vi "PathDrawerMain.vi"() -> ()   [LabVIEW 2018]
uses:
  StartingPositions.ctl
  Dawgma Programming Library/Controls/PurePursuit/PathFileData.ctl
  Dawgma Programming Library/Controls/PurePursuit/RobotNeededPathData.ctl
  <vilib>/Utility/miscctls.llb/LVBoundsTypeDef.ctl
  Robot-Project/Configuration/Constants.vi
panel:
  in  "NoUpdate":bool
  out "PathsStorage":T1[](array[typedef])=[{"RobotNeeded"={"Path"=[{67.51826792963463, 204.30852503382948}, {73.33752695702532, 204.17640783242763}, {79.12917348553499, 204.07996681682357}, {84.86117778762187, 204.06061787570727}, {90.49184817844007, 204.17225057986516}, {95.96307089902717, 204.48997502749893}, {101.19090415563274, 205.12228366964248}, {106.05199464247043, 206.2286051295332}, {110.36361644562574, 208.04511161169543}, {114.37172578385798, 210.89248691926605}, {118.17642408641785, 214.43024981480622}, {121.84478802267412, 218.4296155778484}, {125.42197657870013, 222.73663853194364}, {128.93822516173634, 227.24710298781127}, {132.4139659676452, 231.88974137154145}, {135.8631515190472, 236.6147503980893}, {139.2952430485304, 241.3855785202741}, {142.71714395845063, 246.1731860201357}, {146.13394637043862, 250.9511479319172}, {149.5499982146016, 255.691538218544}, {152.9695484837296, 260.36036298292}, {156.39736200192732, 264.9119963112372}, {159.8395350266317, 269.28183564054643}, {163.30451800782737, 273.375872369032}, {166.80445999957857, 277.0554498679603}, {170.3571607758867, 280.1148018612651}, {174.375619494585, 282.81240477743506}, {178.60376106475013, 285.2362954814753}, {182.8194665712848, 287.43019005020165}, {186.79860760663416, 289.40056942324793}, {190.27875507442488, 291.11772665764545}], "MaxVel"=150.0, "MaxAccel"=150.0, "Backwards?"=FALSE, "PointSpacing"=6.0, "LookaheadDist"=17.0, "Speed/Curve"=3.0, "SlowDistanceAtEnd"=0.0, "SlowSpeed"=15.0, "MaxDeAccel"=120.0}, "Meta"={"Path (px)"=[{97, 141}, {148, 144}, {211, 52}, {237, 42}], "RobotWidth"=33.0, "RobotLength"=38.5, "CenterOfRotYOffset"=19.5, "Roundedness"=0.8606565656565657, "StartingPositionPreset"=0}}] {"RobotNeeded"."SlowSpeed" format="%#_13g"; "RobotNeeded"."SlowDistanceAtEnd" format="%#_13g"; "RobotNeeded"."Speed/Curve" format="%#_13g"}
  in  "Tab Control":enum32{"Path", "Load/Save"}(tab)
  in  "SetStart":bool
  in  "Deaccel":dbl=120.0 format="%#_13g"
  in  "SlowSpeed":dbl=15.0 format="%#_13g"
  in  "SlowDistanceAtEnd":dbl format="%#_13g"
  in  "Speed/Curve":dbl=3.0 format="%#_13g"
  in  "DriveBackwards?":bool
  in  "Lookahead":dbl=17.0
  in  "Points (in)":cluster{dbl, dbl}[](array[cluster])=[{67.51826792963463, 204.30852503382948}, {73.33752695702532, 204.17640783242763}, {79.12917348553499, 204.07996681682357}, {84.86117778762187, 204.06061787570727}, {90.49184817844007, 204.17225057986516}, {95.96307089902717, 204.48997502749893}, {101.19090415563274, 205.12228366964248}, {106.05199464247043, 206.2286051295332}, {110.36361644562574, 208.04511161169543}, {114.37172578385798, 210.89248691926605}, {118.17642408641785, 214.43024981480622}, {121.84478802267412, 218.4296155778484}, {125.42197657870013, 222.73663853194364}, {128.93822516173634, 227.24710298781127}, {132.4139659676452, 231.88974137154145}, {135.8631515190472, 236.6147503980893}, {139.2952430485304, 241.3855785202741}, {142.71714395845063, 246.1731860201357}, {146.13394637043862, 250.9511479319172}, {149.5499982146016, 255.691538218544}, {152.9695484837296, 260.36036298292}, {156.39736200192732, 264.9119963112372}, {159.8395350266317, 269.28183564054643}, {163.30451800782737, 273.375872369032}, {166.80445999957857, 277.0554498679603}, {170.3571607758867, 280.1148018612651}, {174.375619494585, 282.81240477743506}, {178.60376106475013, 285.2362954814753}, {182.8194665712848, 287.43019005020165}, {186.79860760663416, 289.40056942324793}, {190.27875507442488, 291.11772665764545}]
  out "Points (px)":cluster{dbl, dbl}[](array[cluster])=[{97.0, 141.0}, {148.0, 144.0}, {211.0, 52.0}, {237.0, 42.0}]
  in  "Roundedness":dbl(slide)=0.8606565656565657 scale=0.6..0.997
  in  "PointSpacing":dbl=6.0 min=1.0 format="%#_13g"
  in  "Flip Path":bool
  in  "MaxVel":dbl=150.0 format="%#_13g"
  in  "Accel":dbl=150.0 format="%#_13g"
  in  "StartingPosition":T3
  in  "Multiple Paths":i32(listbox)
  in  "ExportAllToRobot":bool
  in  "LocalTempPaths":i32(listbox)
  out "standard output":string
  in  "SaveToLocal":bool
  in  "LoadFromLocal":bool
  in  "ExportToRobot":bool
  in  "LoadAllFromRobot":bool
  in  "LocalPaths":i32(listbox)
  out "standard error":string="NI Linux Real-Time (run mode)\n\nLog in with your NI-Auth credentials.\n\n"
  in  "LocalFileNames":string[](array[string])=["1LL.txt", "3RR.txt"]
  out "Path Drawer":T4(plugin-control)
  # "(Double Click)"
  # "INSTRUCTIONS"
  # "The red line is the path that the robot recieves. Everything else is to help create that path\n\nUse the multi-line tool to draw a path. Double click to stop drawing.\nHover over a node and press backspace to remove it.\nPress I to insert a new node (at the end of the path only, for now)\n\nUse the contols to input robot width, height, and center of rotation offset,\nHow far apart the points in the \"real world units\" path are,\nWhether the robot travels on the left or right of your green lines, and\nthe roundedness of the path. (Note: point spacing affects roundedness)\n\nYou can manually edit the green node's location in the path with the Points array,\nor drag the nodes on the image\n\nPress Export To File and enter the file name (no extension) to save the path to a file in the\nThisVIsDirectory\\Paths\\ folder\n\nIf you acidentally clear your path press Z quickly to get it back"
  # "Responses of CMDs run"
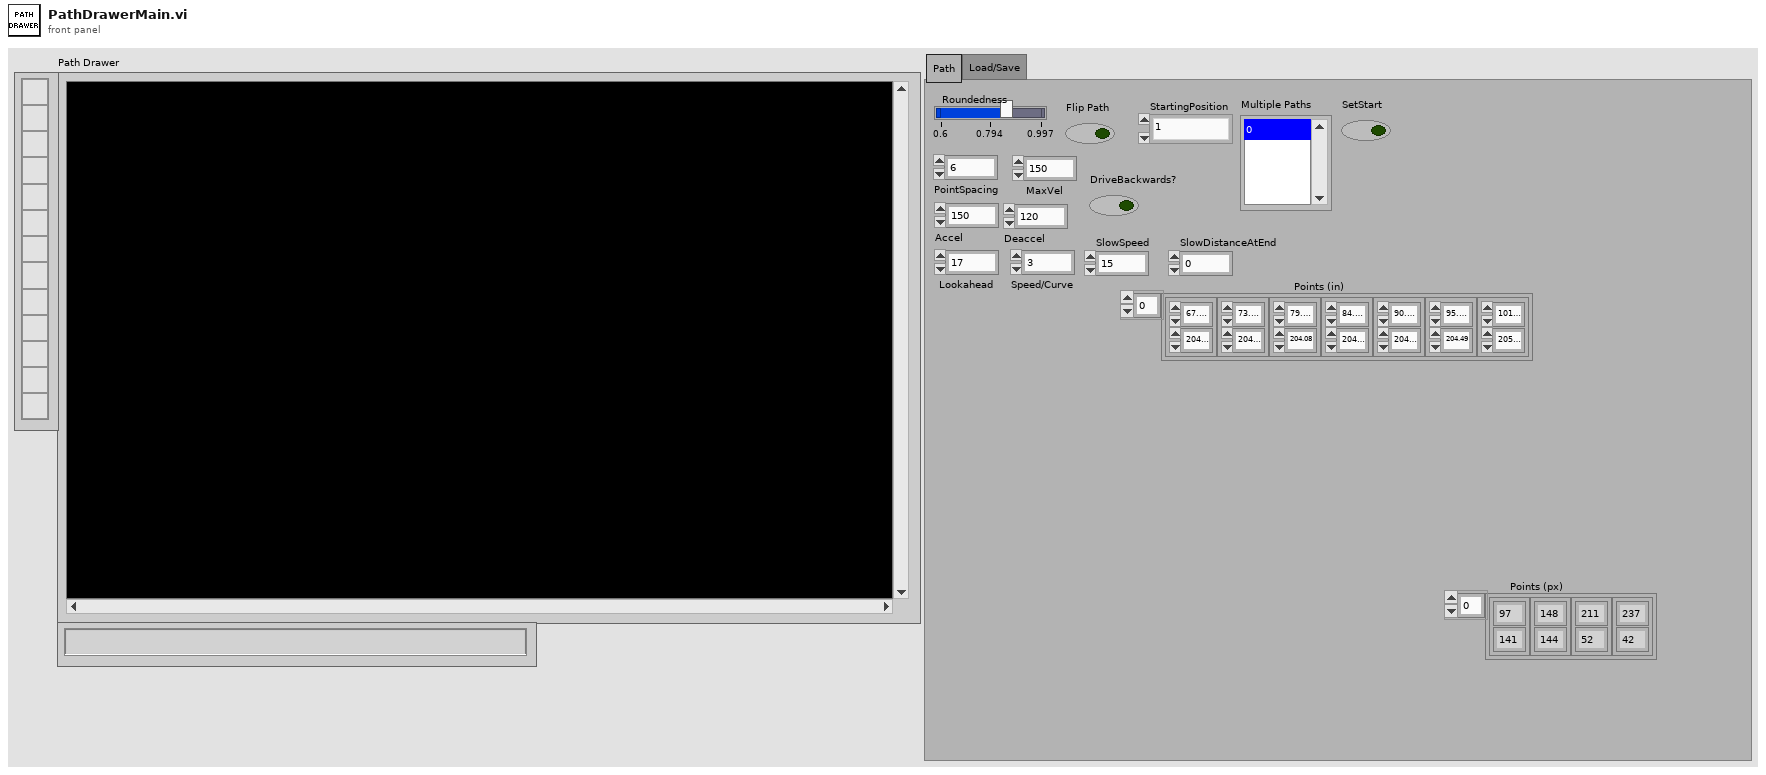
[diagram p1: front panel]
types:
  T1 = typedef "PathFileData.ctl" = cluster{"RobotNeeded":T2, "Meta":cluster{"Path (px)":cluster{i32, i32}[], "RobotWidth":dbl, "RobotLength":dbl, "CenterOfRotYOffset":dbl, "Roundedness":dbl, "StartingPositionPreset":u32}}
  T2 = typedef "RobotNeededPathData.ctl" = cluster{"Path":cluster{dbl, dbl}[], "MaxVel":dbl, "MaxAccel":dbl, "Backwards?":bool, "PointSpacing":dbl, "LookaheadDist":dbl, "Speed/Curve":dbl, "SlowDistanceAtEnd":dbl, "SlowSpeed":dbl, "MaxDeAccel":dbl}
  T3 = typedef "StartingPositions.ctl" = enum16{"1", "2", "3", "4", "5", "No Preset"}
  T4 = typedef "IMAQ Image.ctl" = refnum<image>
  T5 = typedef "Image Type" = u32
  T6 = enum16{"open", "replace", "create", "open or create", "replace or create", "replace or create with confirmation"}
  T7 = typedef "LVBoundsTypeDef.ctl" = cluster{"Width":u32, "Height":u32}
  T8 = cluster{"Global Rectangle":i32[], "Contours":cluster{"Contour Type":u32, "ROI Type":u32, "Points":i32[]}[]}
  T9 = cluster{"Contour Type":u32, "ROI Type":u32, "Points":i32[]}[]
  T10 = cluster{"Contour Type":u32, "ROI Type":u32, "Points":i32[]}
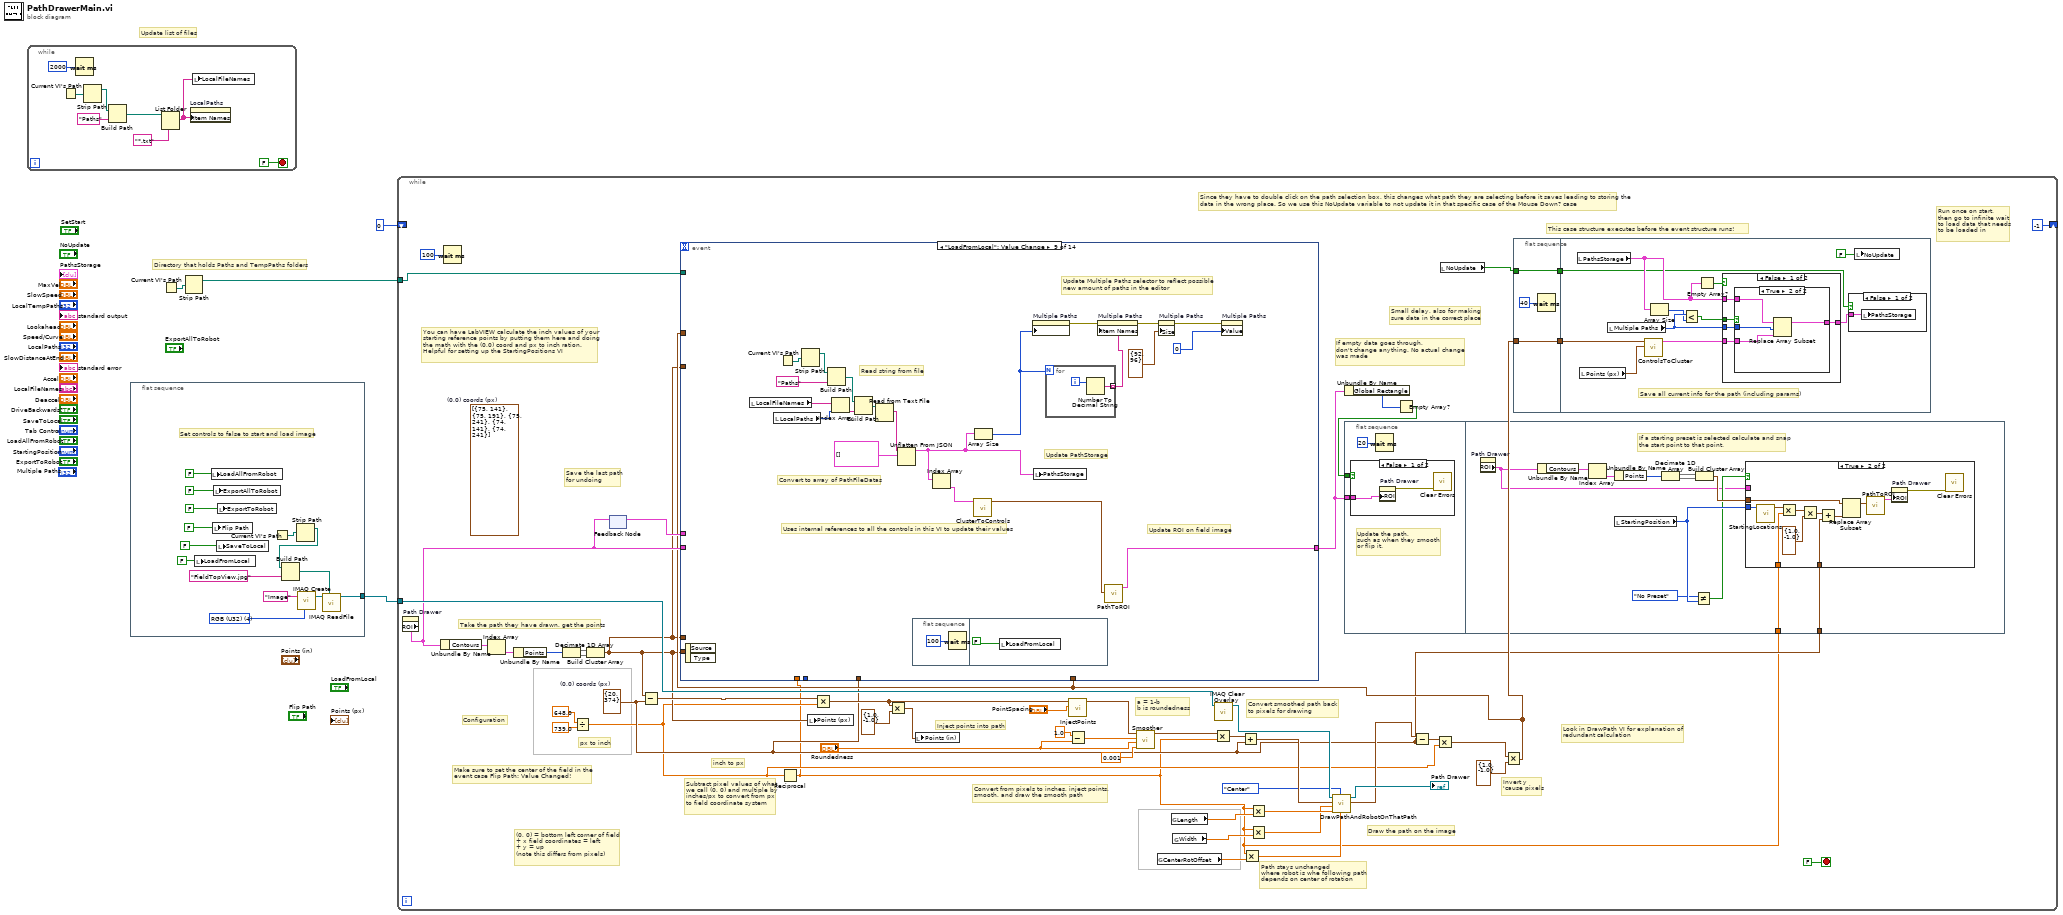
[diagram p0: block diagram]
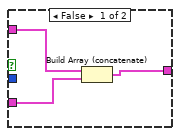
[diagram p3: hidden frame]
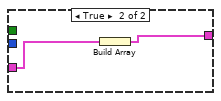
[diagram p4: hidden frame]
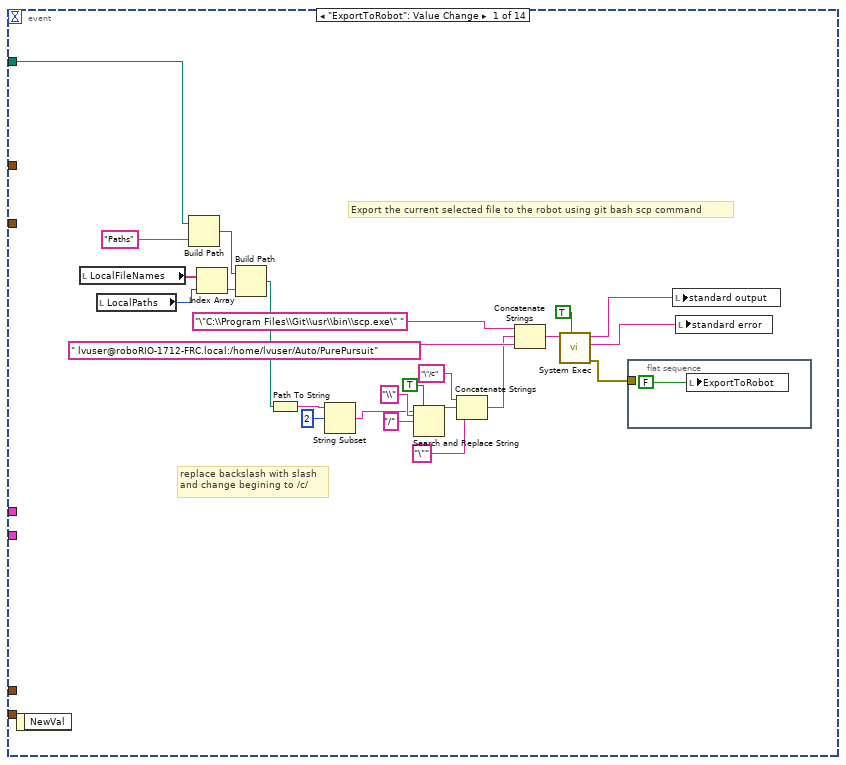
[diagram p7: hidden frame]
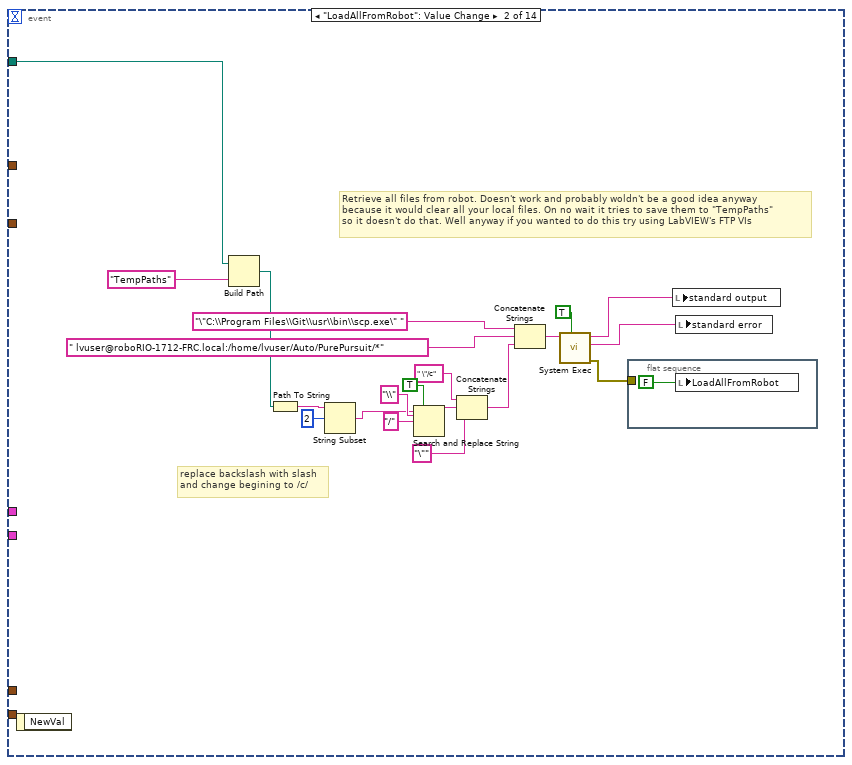
[diagram p8: hidden frame]
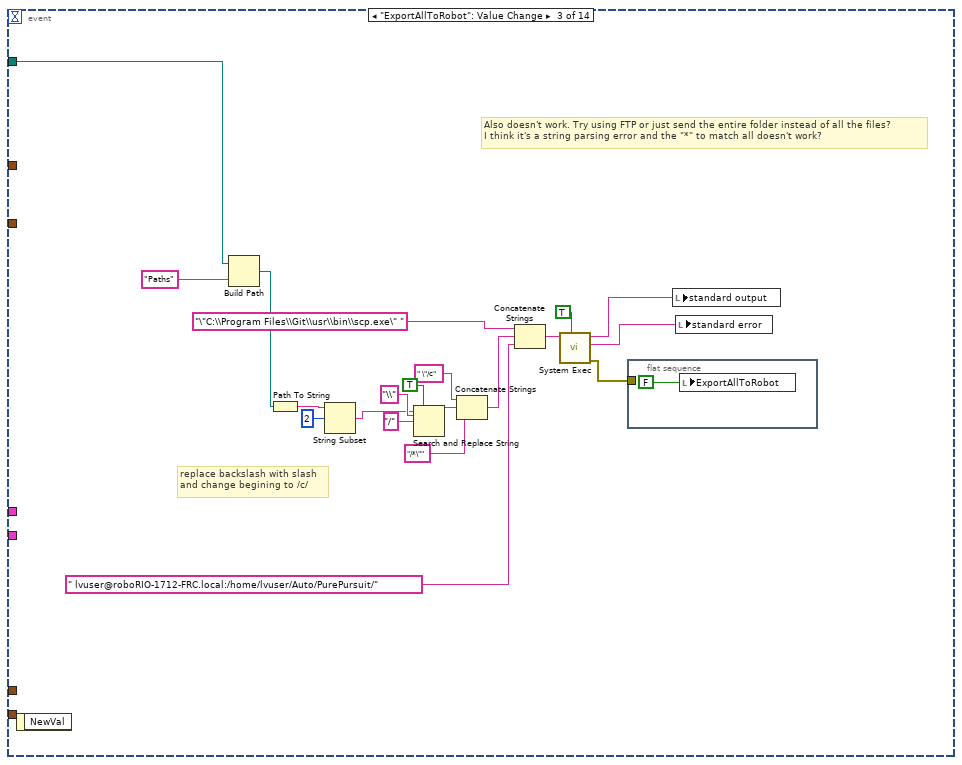
[diagram p9: hidden frame]
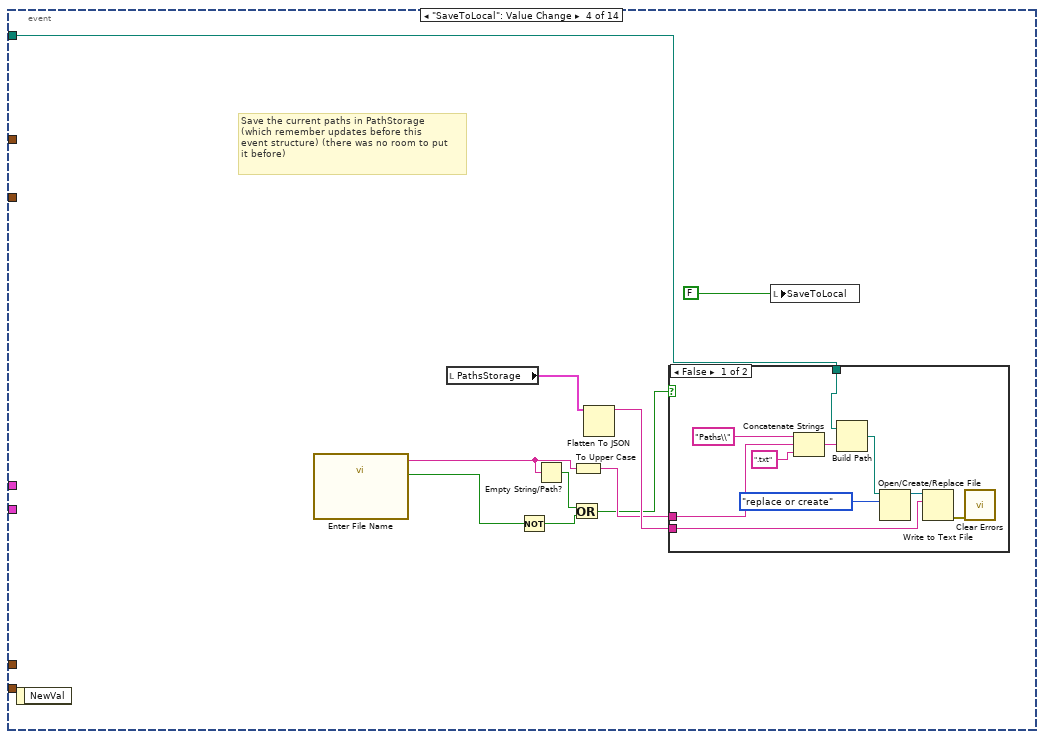
[diagram p10: hidden frame]
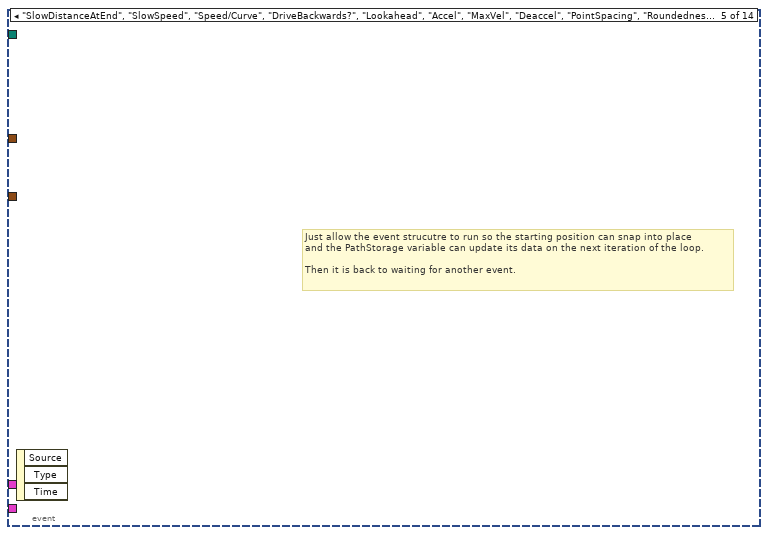
[diagram p12: hidden frame]
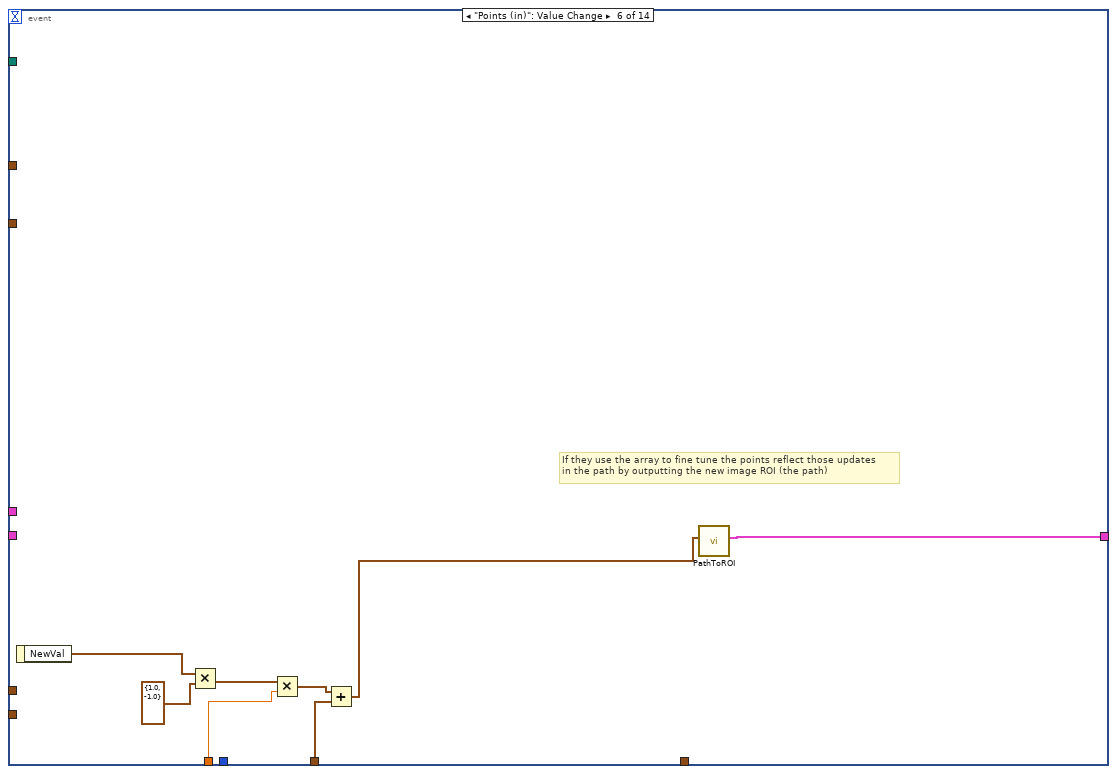
[diagram p13: hidden frame]
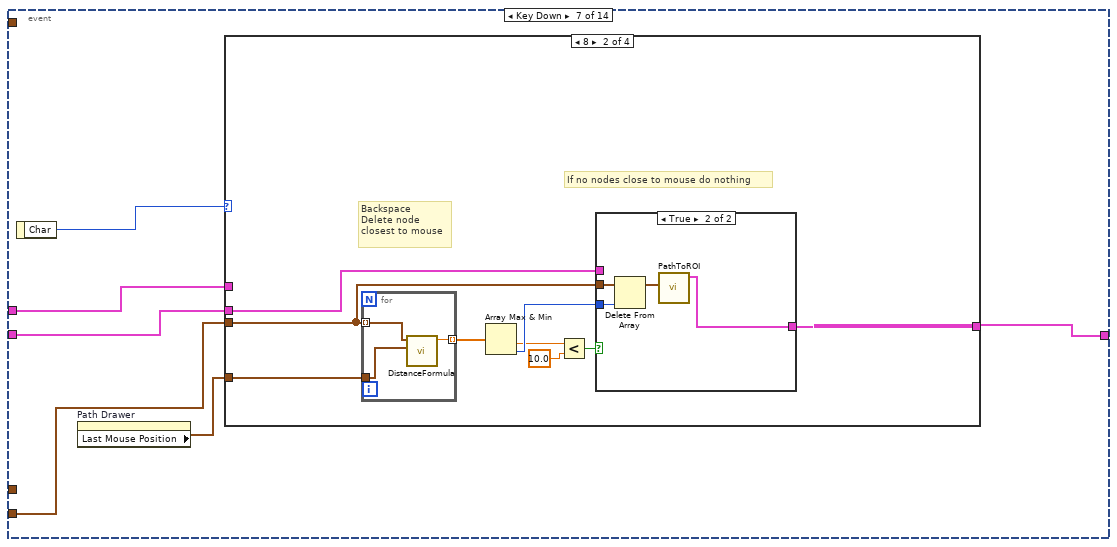
[diagram p14: hidden frame]
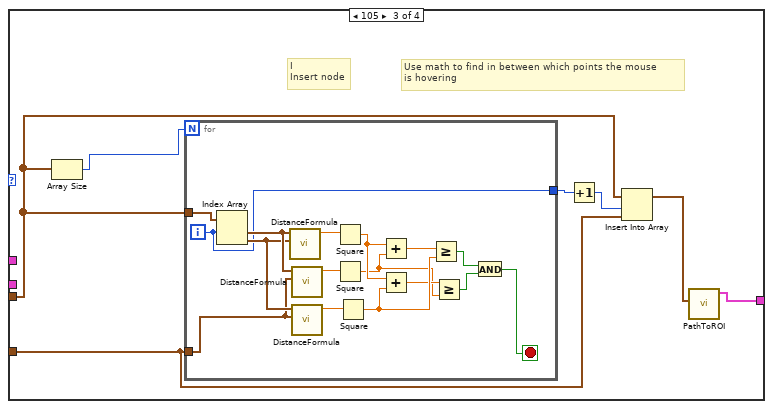
[diagram p17: hidden frame]
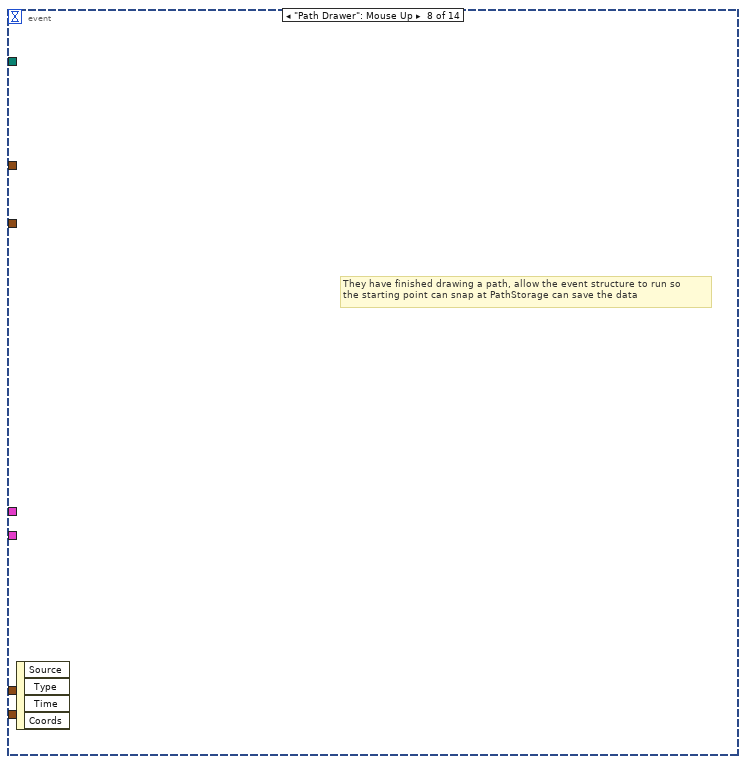
[diagram p19: hidden frame]
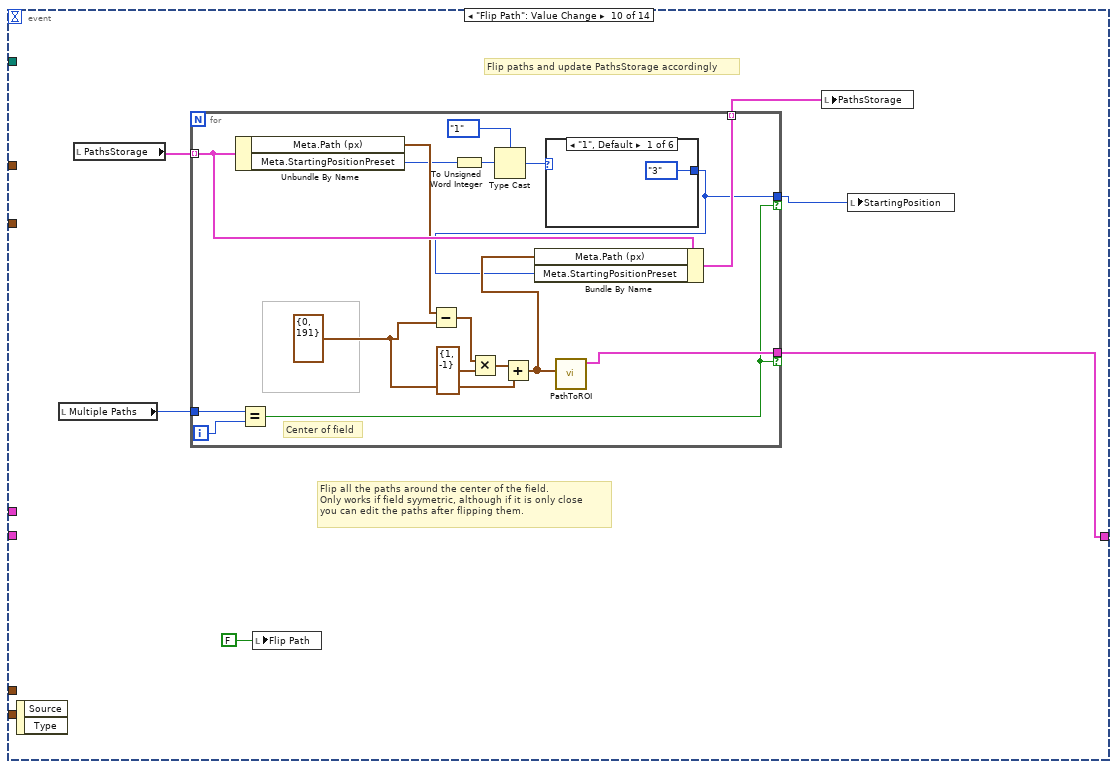
[diagram p20: hidden frame]
diagram:
  # "Update list of files"
  # "Directory that holds Paths and TempPaths folders"
  n1 = while {
    stop <- FALSE stop-if-true
    n2 = Current VI's Path() -> (path=w7:path)
    n3 = Wait (ms)(milliseconds to wait=u32 2000) -> ()  [unwired: 1 out]
    n4 = Strip Path(path=w7) -> (stripped path=w6:path)  [unwired: 1 out]
    n5 = Build Path(base path=w6, name or relative path="Paths") -> (appended path=w9:path)
    n6 = List Folder(path=w9, pattern="*.txt") -> (filenames=w11:string[])  [unwired: 2 in, 3 out]
    n7 = property on="LocalPaths" class="LstBox (strict)"("Item Names"=w11) -> ()  [unwired: 2 in, 2 out]
    n8 = local write "LocalFileNames"(w11) -> ()
  }
  n9 = flat-sequence {
    tunnel: [w21] -> w4
    frame #0 {
      w23 = T5 4 items=["Grayscale (U8)", "Grayscale (I16)", "Grayscale (SGL)", "Complex (CSG)", "RGB (U32)", "HSL (U32)", "RGB (U64)", "Grayscale (U16)"] ("Image Type")
      # "Set controls to false to start and load image"
      n10 = local write "LoadFromLocal"(FALSE ("Export To File")) -> ()
      n11 = local write "LoadAllFromRobot"(FALSE ("Export To File")) -> ()
      n12 = local write "Flip Path"(FALSE ("Export To File")) -> ()
      n13 = local write "ExportAllToRobot"(FALSE ("Export To File")) -> ()
      n14 = local write "SaveToLocal"(FALSE ("Export To File")) -> ()
      n15 = local write "ExportToRobot"(FALSE ("Export To File")) -> ()
      n16 = Current VI's Path() -> (path=w16:path)
      n17 = Strip Path(path=w16) -> (stripped path=w15:path)  [unwired: 1 out]
      n18 = Build Path(base path=w15, name or relative path="FieldTopView.jpg") -> (appended path=w25:path)
      n19 = call "IMAQ Create"("Image Name"="Image", "Image Type"=w23) -> ("New Image"=w22:T4)  [unwired: 3 in, 1 out]
      n20 = call "IMAQ ReadFile"("File Path"=w25, "Image"=w22) -> ("Image Out"=w21:T4)  [unwired: 5 in, 4 out]
    }
  }
  n21 = Current VI's Path() -> (path=w3:path)
  n22 = Strip Path(path=w3) -> (stripped path=w2:path)  [unwired: 1 out]
  n23 = while {
    tunnel: w4 -> [w71]
    tunnel: w2 -> [w46]
    shift-right: [-1] -> _
    shift-left: 0 -> [_]
    stop <- FALSE stop-if-true
    (unwired) cluster{i32, i32}[] [{75, 141}, {75, 191}, {75, 241}, {74, 141}, {74, 241}]  # (0,0) coords (px)
    w29 = cluster{i32, i32} {20, 374}  # (0,0) coords (px)
    # "You can have LabVIEW calculate the inch values of your\nstarting reference points by putting them here and doing\nthe math with the (0,0) coord and px to inch ration.\nHelpful for setting up the StartingPositions VI"
    # "Small delay, also for making\nsure data in the correct place"
    # "Since they have to double click on the path selection box, this changes what path they are selecting before it saves leading to storing the\ndata in the wrong place. So we use this NoUpdate variable to not update it in that specific case of the Mouse Down? case"
    # "This case structure executes before the event structure runs!"
    # "Look in DrawPath VI for explanation of \nredundant calculation"
    # "Draw the path on the image"
    # "a = 1-b\nb is roundedness"
    # "Inject points into path"
    # "(0, 0) = bottom left corner of field\n+ x field coordinates = left\n+ y = up\n(note this differs from pixels)"
    # "Take the path they have drawn, get the points"
    # "Save the last path\nfor undoing"
    # "Make sure to set the center of the field in the\nevent case Flip Path: Value Changed!"
    # "inch to px"
    # "px to inch"
    # "Configuration"
    # "Run once on start,\nthen go to infinite wait\nto load data that needs\nto be loaded in"
    # "Invert y\n'cause pixels"
    # "Path stays unchanged\nwhere robot is whe following path\ndepends on center of rotation"
    # "Convert smoothed path back\nto pixels for drawing"
    # "If empty data goes through,\ndon't change anything. No actual change\nwas made"
    # "Convert from pixels to inches, inject points,\nsmooth, and draw the smooth path"
    # "Subtract pixel values of what\nwe call (0, 0) and multiple by\ninches/px to convert from px\nto field coordinate system"
    n24 = property on="Path Drawer" class="ImageControl"() -> ("ROI"=w48:T8)  [unwired: 2 in, 2 out]
    n25 = Unbundle By Name(w48) -> ("Contours"=w77:T9)
    n26 = Wait (ms)(milliseconds to wait=u32 100) -> ()  [unwired: 1 out]
    n27 = Index Array(array=w77) -> (element=w72:T10)  [unwired: 1 in]
    n28 = Unbundle By Name(w72) -> ("Points"=w66:i32[])
    n29 = Decimate 1D Array(w66) -> (w76:i32[], w75:i32[])
    n30 = Divide(x=648.0, y=739.0) -> (x/y=w28:dbl)
    n31 = Build Cluster Array(w76, w75) -> (w33:cluster{i32, i32}[])
    n32 = feedback-in #1(w48) -> ()
    n33 = feedback #1() -> (w58:T8)  [unwired: 1 in]
    n34 = Subtract(x=w33, y=w29) -> (x-y=w67:cluster{i32, i32}[])
    n35 = Reciprocal(x=w28) -> (1/x=w27:dbl)
    n36 = local write "Points (px)"(w33) -> ()
    n37 = Multiply(x=w67, y=w28) -> (x*y=w31:cluster{dbl, dbl}[])
    n38 = Multiply(x=w31, y=cluster{dbl, dbl} {1.0, -1.0}) -> (x*y=w30:cluster{dbl, dbl}[])
    n39 = local write "Points (in)"(w30) -> ()
    n40 = call "InjectPoints.vi"("Distance"="PointSpacing", "Path"=w31) -> ("Path out"=w69:cluster{dbl, dbl}[])  [unwired: 9 in]
    n41 = Subtract(x=1.0, y="Roundedness") -> (x-y=w64:dbl)
    n42 = call "Smoother.vi"("tolerance"=0.001, "B"="Roundedness", "A"=w64, "Path"=w69) -> ("SmoothPath"=w60:cluster{dbl, dbl}[])  [unwired: 7 in]
    n43 = global read "Constants.vi" "CenterRotOffset"() -> (w34:dbl)
    n44 = global read "Constants.vi" "Length"() -> (w36:dbl)
    n45 = global read "Constants.vi" "Width"() -> (w35:dbl)
    n46 = Multiply(x=w60, y=w27) -> (x*y=w68:cluster{dbl, dbl}[])
    n47 = call "IMAQ Clear Overlay"("Image"=w71) -> ("Image Out"=w54:T4)  [unwired: 9 in, 1 out]
    n48 = Add(x=w68, y=w29) -> (x+y=w53:cluster{dbl, dbl}[])
    n49 = Multiply(x=w27, y=w34) -> (x*y=w43:dbl)
    n50 = Multiply(x=w27, y=w36) -> (x*y=w52:dbl)
    n51 = Multiply(x=w27, y=w35) -> (x*y=w44:dbl)
    n52 = call "DrawPathAndRobotOnThatPath.vi"("CenterOfRotYOffset (px)"=w43, "PathMode"=enum16{"Left", "Right", "Center"}."Center", "RobotLength (px)"=w52, "RobotWidth (px)"=w44, "Path (px)"=w53, "Image In"=w54) -> ("NewPath (px)"=w55:cluster{dbl, dbl}[], "Image Out"=→"Path Drawer":T4)  [unwired: 4 in]
    n53 = flat-sequence {
      tunnel: w47 -> [w109]
      tunnel: w45 -> [w108]
      tunnel: w27 -> [w114]
      tunnel: w29 -> [w113]
      frame #0 {
        # "Update the path,\nsuch as when they smooth\nor flip it."
        n54 = case shown="False" w108 {
          tunnel: w109 -> [w110 _]
          frame False {
            n55 = property on="Path Drawer" class="ImageControl"("ROI"=w110) -> (error out=w111:errorcluster)  [unwired: 2 in, 1 out]
            n56 = call <vilib>:"Clear Errors.vi"("error in (no error)"=w111) -> ()  [unwired: 5 in, 2 out]
          }
          frame True {
          }
        }
        n57 = Wait (ms)(milliseconds to wait=u32 20) -> ()  [unwired: 1 out]
      }
      frame #1 {
        # "If a starting preset is selected calculate and snap\nthe start point to that point."
        n58 = property on="Path Drawer" class="ImageControl"() -> ("ROI"=w115:T8)  [unwired: 2 in, 2 out]
        n59 = Unbundle By Name(w115) -> ("Contours"=w118:T9)
        n60 = Index Array(array=w118) -> (element=w121:T10)  [unwired: 1 in]
        n61 = Unbundle By Name(w121) -> ("Points"=w122:i32[])
        n62 = local read "StartingPosition"() -> (w123:T3)
        n63 = Decimate 1D Array(w122) -> (w119:i32[], w120:i32[])
        n64 = Not Equal?(x=StartingPositions."No Preset" ("StartingPosition"), y=w123) -> (x != y?=w116:bool)
        n65 = Build Cluster Array(w119, w120) -> (w117:cluster{i32, i32}[])
        n66 = case shown="True" w116 {
          tunnel: w115 -> [_ _]
          tunnel: w117 -> [_ w134]
          tunnel: w123 -> [_ w133]
          tunnel: w114 -> [_ w129]
          tunnel: w113 -> [_ w127]
          frame False {
          }
          frame True {
            n67 = call "StartingLocations.vi"("Index"=w133) -> ("Location"=w130:cluster{dbl, dbl})  [unwired: 10 in]
            n68 = Multiply(x=w130, y=w129) -> (x*y=w126:cluster{dbl, dbl})
            n69 = Multiply(x=w126, y=cluster{dbl, dbl} {1.0, -1.0}) -> (x*y=w124:cluster{dbl, dbl})
            n70 = Add(x=w124, y=w127) -> (x+y=w128:cluster{dbl, dbl})
            n71 = Replace Array Subset(array=w134, new element=w128) -> (w135:cluster{i32, i32}[])  [unwired: 1 in]
            n72 = call "PathToROI.vi"("Path In"=w135) -> ("ROI Out"=w131:T8)  [unwired: 10 in]
            n73 = property on="Path Drawer" class="ImageControl"("ROI"=w131) -> (error out=w132:errorcluster)  [unwired: 2 in, 1 out]
            n74 = call <vilib>:"Clear Errors.vi"("error in (no error)"=w132) -> ()  [unwired: 5 in, 2 out]
          }
        }
      }
    }
    n75 = Subtract(x=w55, y=w29) -> (x-y=w59:cluster{dbl, dbl}[])
    n76 = Multiply(x=w59, y=w28) -> (x*y=w50:cluster{dbl, dbl}[])
    n77 = local read "NoUpdate"() -> (w37:bool)
    n78 = Multiply(x=w50, y=cluster{dbl, dbl} {1.0, -1.0}) -> (x*y=w40:cluster{dbl, dbl}[])
    n79 = event shown="[8] \"LoadFromLocal\": Value Change" {
      selector: _ -> [_ _ _ _ _ _ _ _ _ _ _ _ _ _]
      dyn-events: _ -> [_ _ _ _ _ _ _ _ _ _ _ _ _ _]
      timeout: _ -> [_ _ _ _ _ _ _ _ _ _ _ _ _ _]
      tunnel: w48 -> [_ _ _ _ _ _ w236 _ _ _ _ _ w346 w407]
      tunnel: [_ _ _ _ _ w230 w233 _ w298 w307 w334 _ w345 w408] -> w47
      tunnel: w40 -> [_ _ _ _ _ _ _ _ _ _ _ _ _ _]
      tunnel: w58 -> [_ _ _ _ _ _ w232 _ _ _ _ _ _ _]
      tunnel: w33 -> [_ _ _ _ _ _ w231 _ _ _ _ _ _ _]
      tunnel: w33 -> [_ _ _ _ _ _ _ _ _ _ _ _ _ _]
      tunnel: w40 -> [_ _ _ _ _ _ _ _ _ _ _ _ _ _]
      tunnel: w46 -> [w136 w161 w182 w205 _ _ _ _ _ _ _ _ _ _]
      tunnel: [_ _ _ _ _ _ _ _ _ _ w333 _ _ _] -> _
      tunnel: w33 -> [_ _ _ _ _ _ _ _ _ _ _ _ _ _]
      tunnel: w27 -> [_ _ _ _ _ w227 _ _ _ _ _ _ _ _]
      tunnel: w29 -> [_ _ _ _ _ w224 _ _ _ _ _ _ _ _]
      event "ExportToRobot": Value Change {
        # "Export the current selected file to the robot using git bash scp command"
        # "replace backslash with slash\nand change begining to /c/"
        n80 = event-data() -> ()  [unwired: 1 in, 1 out]
        n81 = local read "LocalFileNames"() -> (w143:string[])
        n82 = local read "LocalPaths"() -> (w144:i32)
        n83 = Build Path(base path=w136, name or relative path="Paths") -> (appended path=w146:path)
        n84 = Index Array(array=w143, index=w144) -> (element=w145:string)
        n85 = Build Path(base path=w146, name or relative path=w145) -> (appended path=w141:path)
        n86 = Path To String(path=w141) -> (string=w152:string)
        n87 = String Subset(string=w152, offset (0)=2) -> (substring=w150:string)  [unwired: 1 in]
        n88 = Search and Replace String(replace all?=TRUE ("replace all? (F)"), input string=w150, search string="\\", replace string="/" ("replace string (\"\")")) -> (result string=w149:string)  [unwired: 4 in, 3 out]
        n89 = Concatenate Strings("\"/c" ("string"), w149, "\"" ("string")) -> (w147:string)
        n90 = Concatenate Strings("\"C:\\Program Files\\Git\\usr\\bin\\scp.exe\" " ("command line"), w147, " lvuser@roboRIO-1712-FRC.local:/home/lvuser/Auto/PurePursuit" ("string")) -> (w156:string)
        n91 = call <vilib>:"System Exec.vi"("wait until completion? (T)"=TRUE, "command line"=w156) -> ("error out"=w139:errorcluster, "standard error"=w137:string, "standard output"=w138:string)  [unwired: 6 in, 1 out]
        n92 = flat-sequence {
          tunnel: w139 -> [_]
          frame #0 {
            n93 = local write "ExportToRobot"(FALSE ("Export To File")) -> ()
          }
        }
        n94 = local write "standard output"(w138) -> ()
        n95 = local write "standard error"(w137) -> ()
      }
      event "LoadAllFromRobot": Value Change {
        # "Retrieve all files from robot. Doesn't work and probably woldn't be a good idea anyway\nbecause it would clear all your local files. On no wait it tries to save them to \"TempPaths\"\nso it doesn't do that. Well anyway if you wanted to do this try using LabVIEW's FTP VIs"
        # "replace backslash with slash\nand change begining to /c/"
        n96 = event-data() -> ()  [unwired: 1 in, 1 out]
        n97 = Build Path(base path=w161, name or relative path="TempPaths") -> (appended path=w164:path)
        n98 = Path To String(path=w164) -> (string=w174:string)
        n99 = String Subset(string=w174, offset (0)=2) -> (substring=w172:string)  [unwired: 1 in]
        n100 = Search and Replace String(replace all?=TRUE ("replace all? (F)"), input string=w172, search string="\\", replace string="/" ("replace string (\"\")")) -> (result string=w171:string)  [unwired: 4 in, 3 out]
        n101 = Concatenate Strings(" \"/c" ("string"), w171, "\"" ("string")) -> (w162:string)
        n102 = Concatenate Strings("\"C:\\Program Files\\Git\\usr\\bin\\scp.exe\" " ("command line"), " lvuser@roboRIO-1712-FRC.local:/home/lvuser/Auto/PurePursuit/*" ("string"), w162) -> (w178:string)
        n103 = call <vilib>:"System Exec.vi"("wait until completion? (T)"=TRUE, "command line"=w178) -> ("error out"=w167:errorcluster, "standard error"=w165:string, "standard output"=w166:string)  [unwired: 6 in, 1 out]
        n104 = flat-sequence {
          tunnel: w167 -> [_]
          frame #0 {
            n105 = local write "LoadAllFromRobot"(FALSE ("Export To File")) -> ()
          }
        }
        n106 = local write "standard output"(w166) -> ()
        n107 = local write "standard error"(w165) -> ()
      }
      event "ExportAllToRobot": Value Change {
        # "Also doesn't work. Try using FTP or just send the entire folder instead of all the files?\nI think it's a string parsing error and the \"*\" to match all doesn't work?"
        # "replace backslash with slash\nand change begining to /c/"
        n108 = event-data() -> ()  [unwired: 1 in, 1 out]
        n109 = Build Path(base path=w182, name or relative path="Paths") -> (appended path=w185:path)
        n110 = Path To String(path=w185) -> (string=w195:string)
        n111 = String Subset(string=w195, offset (0)=2) -> (substring=w193:string)  [unwired: 1 in]
        n112 = Search and Replace String(replace all?=TRUE ("replace all? (F)"), input string=w193, search string="\\", replace string="/" ("replace string (\"\")")) -> (result string=w192:string)  [unwired: 4 in, 3 out]
        n113 = Concatenate Strings(" \"/c" ("string"), w192, "/*\"" ("string")) -> (w184:string)
        n114 = Concatenate Strings("\"C:\\Program Files\\Git\\usr\\bin\\scp.exe\" " ("command line"), w184, " lvuser@roboRIO-1712-FRC.local:/home/lvuser/Auto/PurePursuit/" ("string")) -> (w199:string)
        n115 = call <vilib>:"System Exec.vi"("wait until completion? (T)"=TRUE, "command line"=w199) -> ("error out"=w188:errorcluster, "standard error"=w186:string, "standard output"=w187:string)  [unwired: 6 in, 1 out]
        n116 = flat-sequence {
          tunnel: w188 -> [_]
          frame #0 {
            n117 = local write "ExportAllToRobot"(FALSE ("Export To File")) -> ()
          }
        }
        n118 = local write "standard output"(w187) -> ()
        n119 = local write "standard error"(w186) -> ()
      }
      event "SaveToLocal": Value Change {
        # "Save the current paths in PathStorage\n(which remember updates before this\nevent structure) (there was no room to put\nit before)"
        n120 = event-data() -> ()  [unwired: 1 in, 1 out]
        n121 = call "Enter File Name"() -> ("File Name"=w207:string, "Enter"=w209:bool)  [unwired: 17 in, 1 out]
        n122 = local read "PathsStorage"() -> (w203:T1[])
        n123 = Not(x=w209) -> (.not. x?=w208:bool)
        n124 = Empty String/Path?(string/path=w207) -> (empty?=w210:bool)
        n125 = Or(x=w210, y=w208) -> (x .or. y?=w204:bool)
        n126 = To Upper Case(1:w207) -> (0:w206:string)
        n127 = Flatten To JSON(anything=w203) -> (JSON string=w211:string)  [unwired: 2 in, 1 out]
        n128 = case shown="False" w204 {
          tunnel: w206 -> [w218 _]
          tunnel: w211 -> [w217 _]
          tunnel: w205 -> [w213 _]
          frame False {
            n129 = Concatenate Strings("Paths\\" ("name or relative path"), w218, ".txt" ("string")) -> (w222:string)
            n130 = Build Path(base path=w213, name or relative path=w222) -> (appended path=w216:path)
            n131 = Open/Create/Replace File(file path (use dialog)=w216, operation (0:open)=T6."replace or create") -> (refnum out=w215:refnum<file>)  [unwired: 4 in, 2 out]
            n132 = Write to Text File(file (use dialog)=w215, text=w217) -> (error out=w220:errorcluster)  [unwired: 2 in, 2 out]
            n133 = call <vilib>:"Clear Errors.vi"("error in (no error)"=w220) -> ()  [unwired: 5 in, 2 out]
          }
          frame True {
          }
        }
        n134 = local write "SaveToLocal"(FALSE ("Export To File")) -> ()
      }
      event "SlowDistanceAtEnd", "SlowSpeed", "Speed/Curve", "DriveBackwards?", "Lookahead", "Accel", "MaxVel", "Deaccel", "PointSpacing", "Roundedness": Value Change; Mouse Down; Timeout {
        # "Just allow the event strucutre to run so the starting position can snap into place\nand the PathStorage variable can update its data on the next iteration of the loop.\n\nThen it is back to waiting for another event."
        n135 = event-data() -> ()  [unwired: 1 in, 3 out]
      }
      event "Points (in)": Value Change {
        # "If they use the array to fine tune the points reflect those updates\nin the path by outputting the new image ROI (the path)"
        n136 = event-data() -> ("NewVal"=w228:cluster{dbl, dbl}[])  [unwired: 1 in]
        n137 = Multiply(x=w228, y=cluster{dbl, dbl} {1.0, -1.0}) -> (x*y=w226:cluster{dbl, dbl}[])
        n138 = Multiply(x=w226, y=w227) -> (x*y=w225:cluster{dbl, dbl}[])
        n139 = Add(x=w225, y=w224) -> (x+y=w223:cluster{dbl, dbl}[])
        n140 = call "PathToROI.vi"("Path In"=w223) -> ("ROI Out"=w230:T8)  [unwired: 10 in]
      }
      event Key Down {
        n141 = event-data() -> ("Char"=w235:i16)  [unwired: 1 in]
        n142 = property on="Path Drawer" class="ImageControl"() -> ("Last Mouse Position"=w234:cluster{"X":i32, "Y":i32})  [unwired: 2 in, 2 out]
        n143 = case shown="8" w235 {
          tunnel: w236 -> [w237 w246 _ _]
          tunnel: w231 -> [_ w245 w259 _]
          tunnel: w234 -> [_ w239 w260 _]
          tunnel: [w237 w238 w261 w278] -> w233
          tunnel: w232 -> [_ _ _ w278]
          frame 0, Default {
            # "Nothing"
          }
          frame 8 {
            # "If no nodes close to mouse do nothing"
            # "Backspace\nDelete node\nclosest to mouse"
            n144 = for {
              tunnel: w245 -> [w254] mode=indexing
              tunnel: [w253] -> w244 mode=indexing
              tunnel: w239 -> [w252]
              n145 = call "DistanceFormula.vi"("Point 2"=w252, "Point 1"=w254) -> ("Distance"=w253:dbl)  [unwired: 9 in]
            }
            n146 = Array Max & Min(array=w244) -> (min value=w242:dbl, min index (indices)=w243:i32)  [unwired: 2 out]
            n147 = Less?(x=w242, y=10.0) -> (x < y?=w240:bool)
            n148 = case shown="True" w240 {
              tunnel: w243 -> [_ w251]
              tunnel: w245 -> [_ w250]
              tunnel: w246 -> [w247 _]
              tunnel: [w247 w248] -> w238
              frame False {
              }
              frame True {
                n149 = Delete From Array(array=w250, index=w251) -> (array with subset deleted=w249:cluster{i32, i32}[])  [unwired: 1 in, 1 out]
                n150 = call "PathToROI.vi"("Path In"=w249) -> ("ROI Out"=w248:T8)  [unwired: 10 in]
              }
            }
          }
          frame 105 {
            # "Use math to find in between which points the mouse\nis hovering"
            # "I\nInsert node"
            n151 = Array Size(array=w259) -> (size(s)=w255:i32)
            n152 = for {
              N: w255 -> [_]
              tunnel: w259 -> [w277]
              tunnel: w260 -> [w274]
              tunnel: [w262] -> w257
              i -> [w262]
              stop <- w263 stop-if-true
              n153 = Index Array(array=w277, index #1=w262) -> (element #1=w276:cluster{i32, i32}, element #2=w275:cluster{i32, i32})  [unwired: 1 in]
              n154 = call "DistanceFormula.vi"("Point 2"=w275, "Point 1"=w276) -> ("Distance"=w273:dbl)  [unwired: 9 in]
              n155 = call "DistanceFormula.vi"("Point 2"=w274, "Point 1"=w276) -> ("Distance"=w272:dbl)  [unwired: 9 in]
              n156 = call "DistanceFormula.vi"("Point 2"=w274, "Point 1"=w275) -> ("Distance"=w271:dbl)  [unwired: 9 in]
              n157 = Square(x=w273) -> (x^2=w270:dbl)
              n158 = Square(x=w272) -> (x^2=w266:dbl)
              n159 = Square(x=w271) -> (x^2=w268:dbl)
              n160 = Add(x=w270, y=w266) -> (x+y=w269:dbl)
              n161 = Add(x=w270, y=w268) -> (x+y=w267:dbl)
              n162 = Greater Or Equal?(x=w269, y=w268) -> (x >= y?=w265:bool)
              n163 = Greater Or Equal?(x=w267, y=w266) -> (x >= y?=w264:bool)
              n164 = And(x=w265, y=w264) -> (x .and. y?=w263:bool)
            }
            n165 = Increment(x=w257) -> (x+1=w256:i32)
            n166 = Insert Into Array(array=w259, index=w256, new element=w260) -> (w258:cluster{i32, i32}[])
            n167 = call "PathToROI.vi"("Path In"=w258) -> ("ROI Out"=w261:T8)  [unwired: 10 in]
          }
          frame 122 {
            # "Restore last ROI"
            # "Z"
          }
        }
      }
      event "Path Drawer": Mouse Up {
        # "They have finished drawing a path, allow the event structure to run so\nthe starting point can snap at PathStorage can save the data"
        n168 = event-data() -> ()  [unwired: 1 in, 4 out]
      }
      event "LoadFromLocal": Value Change {
        # "Update Multiple Paths selector to reflect possible\nnew amount of paths in the editor"
        # "Update ROI on field image"
        # "Update PathStorage"
        # "Convert to array of PathFileDatas"
        # "Read string from file"
        # "Uses internal references to all the controls in this VI to update their values"
        n169 = event-data() -> ()  [unwired: 1 in, 2 out]
        n170 = local read "LocalFileNames"() -> (w290:string[])
        n171 = local read "LocalPaths"() -> (w291:i32)
        n172 = Current VI's Path() -> (path=w293:path)
        n173 = Strip Path(path=w293) -> (stripped path=w292:path)  [unwired: 1 out]
        n174 = Build Path(base path=w292, name or relative path="Paths") -> (appended path=w296:path)
        n175 = Index Array(array=w290, index=w291) -> (element=w295:string)
        n176 = Build Path(base path=w296, name or relative path=w295) -> (appended path=w294:path)
        n177 = Read from Text File(file (use dialog)=w294) -> (text=w297:string)  [unwired: 3 in, 3 out]
        n178 = Unflatten From JSON(JSON string=w297, type and defaults=T1[] []) -> (value=w286:T1[])  [unwired: 5 in, 1 out]
        n179 = flat-sequence {
          frame #0 {
            n180 = Wait (ms)(milliseconds to wait=u32 100) -> ()  [unwired: 1 out]
          }
          frame #1 {
            n181 = local write "LoadFromLocal"(FALSE ("Export To File")) -> ()
          }
        }
        n182 = Index Array(array=w286) -> (element=w287:T1)  [unwired: 1 in]
        n183 = call "ClusterToControls.vi"("Path File Data"=w287) -> ("Path (px)"=w289:cluster{i32, i32}[])  [unwired: 10 in]
        n184 = Array Size(array=w286) -> (size(s)=w283:i32)
        n185 = property on="Multiple Paths" class="LstBox (strict)"("Number of Rows"=w283) -> (error out=w285:errorcluster)  [unwired: 2 in, 1 out]
        n186 = local write "PathsStorage"(w286) -> ()
        n187 = for {
          N: w283 -> [_]
          tunnel: [w300] -> w281 mode=indexing
          i -> [w301]
          n188 = Number To Decimal String(number=w301) -> (decimal integer string=w300:string)  [unwired: 1 in]
        }
        n189 = property on="Multiple Paths" class="LstBox (strict)"(error in=w285, "Item Names"=w281) -> (error out=w284:errorcluster)  [unwired: 1 in, 1 out]
        n190 = call "PathToROI.vi"("Path In"=w289) -> ("ROI Out"=w298:T8)  [unwired: 10 in]
        n191 = property on="Multiple Paths" class="LstBox (strict)"(error in=w284, "Size"=T7 {"Width"=92, "Height"=96}) -> (error out=w279:errorcluster)  [unwired: 1 in, 1 out]
        n192 = property on="Multiple Paths" class="LstBox (strict)"(error in=w279, "Value"=0 ("Active Row:Active Row Number")) -> ()  [unwired: 1 in, 2 out]
      }
      event "Flip Path": Value Change {
        # "Flip paths and update PathsStorage accordingly"
        # "Flip all the paths around the center of the field. \nOnly works if field syymetric, although if it is only close\nyou can edit the paths after flipping them."
        n193 = event-data() -> ()  [unwired: 1 in, 2 out]
        n194 = local read "Multiple Paths"() -> (w305:i32)
        n195 = local read "PathsStorage"() -> (w308:T1[])
        n196 = for {
          tunnel: w308 -> [w326] mode=indexing
          tunnel: [w321] -> w307 if=w314
          tunnel: [w318] -> w306 mode=indexing
          tunnel: w305 -> [w316]
          tunnel: [w315] -> w304 if=w314
          i -> [w317]
          w323 = cluster{i32, i32} {0, 191}
          # "Center of field"
          n197 = Unbundle By Name(w326) -> ("Meta.Path (px)"=w320:cluster{i32, i32}[], "Meta.StartingPositionPreset"=w310:u32)
          n198 = Equal?(x=w316, y=w317) -> (x = y?=w314:bool)
          n199 = Subtract(x=w320, y=w323) -> (x-y=w325:cluster{i32, i32}[])
          n200 = To Unsigned Word Integer(number=w310) -> (unsigned 16bit integer=w311:u16)
          n201 = Multiply(x=w325, y=cluster{i32, i32} {1, -1}) -> (x*y=w324:cluster{i32, i32}[])
          n202 = Type Cast(type=StartingPositions."1" ("StartingPosition"), x=w311) -> (*(type *) &x=w312:T3)
          n203 = Add(x=w324, y=w323) -> (x+y=w319:cluster{i32, i32}[])
          n204 = case shown="\"1\", Default" w312 {
            tunnel: [StartingPositions."3" ("StartingPosition") StartingPositions."2" ("StartingPosition") StartingPositions."1" ("StartingPosition") StartingPositions."5" ("StartingPosition") StartingPositions."4" ("StartingPosition") StartingPositions."No Preset" ("StartingPosition")] -> w315
            frame "1", Default {
            }
            frame "2" {
            }
            frame "3" {
            }
            frame "4" {
            }
            frame "5" {
            }
            frame "No Preset" {
            }
          }
          n205 = Bundle By Name(cluster=w326, "Meta.Path (px)"=w319, "Meta.StartingPositionPreset"=w315) -> (w318:T1)
          n206 = call "PathToROI.vi"("Path In"=w319) -> ("ROI Out"=w321:T8)  [unwired: 10 in]
        }
        n207 = local write "Flip Path"(FALSE ("Export To File")) -> ()
        n208 = local write "PathsStorage"(w306) -> ()
        n209 = local write "StartingPosition"(w304) -> ()
      }
      event "Multiple Paths": Value Change {
        # "Use references to controls on the front panel\nto update their values"
        # "Load the new path into the editor"
        n210 = event-data() -> ("NewVal"=w333:i32)  [unwired: 1 in, 5 out]
        n211 = local read "Multiple Paths"() -> (w335:i32)
        n212 = local read "PathsStorage"() -> (w336:T1[])
        n213 = Index Array(array=w336, index=w335) -> (element=w338:T1)
        n214 = call "ClusterToControls.vi"("Path File Data"=w338) -> ("Path (px)"=w337:cluster{i32, i32}[])  [unwired: 10 in]
        n215 = call "PathToROI.vi"("Path In"=w337) -> ("ROI Out"=w334:T8)  [unwired: 10 in]
      }
      event "Multiple Paths": Mouse Down? {
        # "2 for right click, 1 for regular click.\nBy turning double click into right click we open the options menu"
        n216 = event-data() -> ("Mods"=w344:cluster{"Double Click":bool, "Menu Key":bool})  [unwired: 1 in, 7 out]
        n217 = Unbundle By Name(w344) -> ("Double Click"=w343:bool)
        n218 = Select(t=u16 2 ("Button"), s=w343, f=u16 1) -> (s? t:f=w340:u16)
        n219 = local write "NoUpdate"(TRUE ("NoUpdate")) -> ()
        n220 = event-data("Button"=w340) -> ()  [unwired: 1 in, 1 out]
      }
      event "Multiple Paths": Shortcut Menu Selection (User) {
        # "Modify Paths Storage accordingly"
        n221 = event-data() -> ("ItemTag"=w349:string)  [unwired: 1 in, 7 out]
        n222 = local read "PathsStorage"() -> (w348:T1[])
        n223 = case shown="\"Clear Paths\"" w349 {
          tunnel: w348 -> [w352 w370 w404]
          tunnel: [w351 w375 w403] -> w347
          tunnel: w346 -> [_ _ _]
          tunnel: [_ w374 w395] -> w345
          frame "New Path", Default {
            # "Make the path a short line\nto start"
            # "Add a new path after the location they clicked"
            n224 = Array Size(array=w352) -> (size(s)=w358:i32)
            n225 = Increment(x=w358) -> (x+1=w365:i32)
            n226 = Decrement(x=w358) -> (x-1=w357:i32)
            n227 = Index Array(array=w352, index=w357) -> (element=w361:T1)
            n228 = Unbundle By Name(w361) -> ("Meta.Path (px)"=w360:cluster{i32, i32}[])
            n229 = for {
              N: w365 -> [_]
              tunnel: [w368] -> w367 mode=indexing
              i -> [w369]
              n230 = Number To Decimal String(number=w369) -> (decimal integer string=w368:string)  [unwired: 1 in]
            }
            n231 = property on="Multiple Paths" class="LstBox (strict)"("Number of Rows"=w365) -> (error out=w364:errorcluster)  [unwired: 2 in, 1 out]
            n232 = Reverse 1D Array(array=w360) -> (reversed array=w359:cluster{i32, i32}[])
            n233 = Index Array(array=w359) -> (element=w356:cluster{i32, i32})  [unwired: 1 in]
            n234 = Add(x=w356, y=cluster{i32, i32} {-60, 0}) -> (x+y=w354:cluster{i32, i32})
            n235 = property on="Multiple Paths" class="LstBox (strict)"(error in=w364, "Item Names"=w367) -> (error out=w363:errorcluster)  [unwired: 1 in, 1 out]
            n236 = Build Array(w356, w354) -> (w353:cluster{i32, i32}[])
            n237 = Bundle By Name(cluster=w361, "Meta.StartingPositionPreset"=StartingPositions."No Preset" ("StartingPosition"), "Meta.Path (px)"=w353) -> (w362:T1)
            n238 = Build Array (concatenate)(w352, w362) -> (w351:T1[])
            n239 = property on="Multiple Paths" class="LstBox (strict)"(error in=w363, "Size"=T7 {"Width"=92, "Height"=96}) -> ()  [unwired: 1 in, 2 out]
          }
          frame "Remove Path" {
            # "Don't remove\nif only one\nleft"
            n240 = Array Size(array=w370) -> (size(s)=w373:i32)
            n241 = Greater?(x=w373, y=1) -> (0:w371:bool)
            n242 = case shown="True" w371 {
              tunnel: [w376 w382] -> w375
              tunnel: [_ w381] -> w374
              tunnel: w370 -> [w376 w379]
              frame False {
              }
              frame True {
                # "Just load the first path in because I was lazy"
                # "Remove the path"
                n243 = local read "Multiple Paths"() -> (w378:i32)
                n244 = Delete From Array(array=w379, length=1, index=w378) -> (array with subset deleted=w382:T1[])  [unwired: 1 out]
                n245 = Index Array(array=w382) -> (element=w380:T1)  [unwired: 1 in]
                n246 = Array Size(array=w382) -> (size(s)=w385:i32)
                n247 = for {
                  N: w385 -> [_]
                  tunnel: [w391] -> w386 mode=indexing
                  i -> [w392]
                  n248 = Number To Decimal String(number=w392) -> (decimal integer string=w391:string)  [unwired: 1 in]
                }
                n249 = property on="Multiple Paths" class="LstBox (strict)"("Number of Rows"=w385) -> (error out=w388:errorcluster)  [unwired: 2 in, 1 out]
                n250 = call "ClusterToControls.vi"("Path File Data"=w380) -> ("Path (px)"=w383:cluster{i32, i32}[])  [unwired: 10 in]
                n251 = call "PathToROI.vi"("Path In"=w383) -> ("ROI Out"=w381:T8)  [unwired: 10 in]
                n252 = property on="Multiple Paths" class="LstBox (strict)"(error in=w388, "Item Names"=w386) -> (error out=w387:errorcluster)  [unwired: 1 in, 1 out]
                n253 = property on="Multiple Paths" class="LstBox (strict)"(error in=w387, "Size"=T7 {"Width"=92, "Height"=96}) -> (error out=w377:errorcluster)  [unwired: 1 in, 1 out]
                n254 = property on="Multiple Paths" class="LstBox (strict)"(error in=w377, "Value"=0 ("Active Row:Active Row Number")) -> ()  [unwired: 1 in, 2 out]
              }
            }
          }
          frame "Clear Paths" {
            w398 = u32 1 ("Number of Rows")
            # "Remove all but the first path"
            # "Keep only first path"
            n255 = for {
              N: w398 -> [_]
              tunnel: [w405] -> w402 mode=indexing
              i -> [w406]
              n256 = Number To Decimal String(number=w406) -> (decimal integer string=w405:string)  [unwired: 1 in]
            }
            n257 = property on="Multiple Paths" class="LstBox (strict)"("Number of Rows"=w398) -> (error out=w401:errorcluster)  [unwired: 2 in, 1 out]
            n258 = Index Array(array=w404) -> (element=w396:T1)  [unwired: 1 in]
            n259 = property on="Multiple Paths" class="LstBox (strict)"(error in=w401, "Item Names"=w402) -> (error out=w400:errorcluster)  [unwired: 1 in, 1 out]
            n260 = call "ClusterToControls.vi"("Path File Data"=w396) -> ("Path (px)"=w397:cluster{i32, i32}[])  [unwired: 10 in]
            n261 = property on="Multiple Paths" class="LstBox (strict)"(error in=w400, "Size"=T7 {"Width"=92, "Height"=96}) -> (error out=w394:errorcluster)  [unwired: 1 in, 1 out]
            n262 = call "PathToROI.vi"("Path In"=w397) -> ("ROI Out"=w395:T8)  [unwired: 10 in]
            n263 = property on="Multiple Paths" class="LstBox (strict)"(error in=w394, "Value"=0 ("Multiple Paths")) -> ()  [unwired: 1 in, 2 out]
            n264 = Build Array(w396) -> (w403:T1[])
          }
        }
        n265 = local write "PathsStorage"(w347) -> ()
      }
      event "SetStart": Value Change {
        # "Sets the start of the current selected path to the end of the previous one"
        n266 = event-data() -> ()  [unwired: 1 in, 6 out]
        n267 = local read "Multiple Paths"() -> (w409:i32)
        n268 = Not Equal To 0?(x=w409) -> (x != 0?=w410:bool)
        n269 = case shown="True" w410 {
          tunnel: w409 -> [_ w415]
          tunnel: [_ w411] -> w408
          tunnel: w407 -> [_ _]
          frame False {
          }
          frame True {
            n270 = Decrement(x=w415) -> (x-1=w424:i32)
            n271 = local read "PathsStorage"() -> (w414:T1[])
            n272 = Index Array(array=w414, index #1=w424, index #2=w415) -> (element #1=w423:T1, element #2=w417:T1)
            n273 = Unbundle By Name(w417) -> ("Meta.Path (px)"=w420:cluster{i32, i32}[])
            n274 = Unbundle By Name(w423) -> ("Meta.Path (px)"=w422:cluster{i32, i32}[])
            n275 = Reverse 1D Array(array=w422) -> (reversed array=w421:cluster{i32, i32}[])
            n276 = Index Array(array=w421) -> (element=w419:cluster{i32, i32})  [unwired: 1 in]
            n277 = Replace Array Subset(array=w420, new element=w419, index=0) -> (w412:cluster{i32, i32}[])
            n278 = Bundle By Name(cluster=w417, "Meta.Path (px)"=w412) -> (w416:T1)
            n279 = Replace Array Subset(array=w414, new element=w416, index=w415) -> (w413:T1[])
            n280 = local write "PathsStorage"(w413) -> ()
            n281 = call "PathToROI.vi"("Path In"=w412) -> ("ROI Out"=w411:T8)  [unwired: 10 in]
          }
        }
        n282 = flat-sequence {
          frame #0 {
            n283 = Wait (ms)(milliseconds to wait=u32 100) -> ()  [unwired: 1 out]
          }
          frame #1 {
            n284 = local write "SetStart"(FALSE ("SetStart")) -> ()
          }
        }
      }
    }
    n285 = Unbundle By Name(w47) -> ("Global Rectangle"=w61:i32[])
    n286 = Empty Array?(array=w61) -> (empty?=w45:bool)
    n287 = flat-sequence {
      tunnel: w37 -> [w79]
      tunnel: w40 -> [w80]
      tunnel: [w80] -> w39
      tunnel: [w79] -> w38
      tunnel: w39 -> [w83]
      tunnel: w38 -> [w82]
      frame #0 {
        n288 = Wait (ms)(milliseconds to wait=u32 40) -> ()  [unwired: 1 out]
      }
      frame #1 {
        # "Save all current info for the path (including params)"
        n289 = local read "PathsStorage"() -> (w85:T1[])
        n290 = local read "Points (px)"() -> (w91:cluster{dbl, dbl}[])
        n291 = local read "Multiple Paths"() -> (w87:i32)
        n292 = call "ControlsToCluster.vi"("Path (px)"=w91, "Path (in)"=w83) -> ("Path File Data"=w89:T1)  [unwired: 9 in]
        n293 = Array Size(array=w85) -> (size(s)=w86:i32)
        n294 = Less?(x=w87, y=w86) -> (x < y?=w90:bool)
        n295 = Empty Array?(array=w85) -> (empty?=w88:bool)
        n296 = case shown="False" w88 {
          tunnel: [w97 w105] -> w84
          tunnel: w87 -> [w96 _]
          tunnel: w90 -> [w95 _]
          tunnel: w89 -> [w94 w106]
          tunnel: w85 -> [w93 _]
          frame False {
            n297 = case shown="True" w95 {
              tunnel: w93 -> [w99 w104]
              tunnel: w94 -> [w100 w102]
              tunnel: [w98 w103] -> w97
              tunnel: w96 -> [_ w101]
              frame False {
                n298 = Build Array (concatenate)(w99, w100) -> (w98:T1[])
              }
              frame True {
                n299 = Replace Array Subset(array=w104, new element=w102, index=w101) -> (w103:T1[])
              }
            }
          }
          frame True {
            n300 = Build Array(w106) -> (w105:T1[])
          }
        }
        n301 = case shown="False" w82 {
          tunnel: w84 -> [w92 _]
          frame False {
            n302 = local write "PathsStorage"(w92) -> ()
          }
          frame True {
          }
        }
        n303 = local write "NoUpdate"(FALSE ("NoUpdate")) -> ()
      }
    }
  }
